vi "nanocal -- nuclear schottky fit -- 2x2 -- V9.vi"() -> ()   [LabVIEW 2021] (continued)
τC\" -> 0.001114108457   ,  \"κ0\" -> 0.000000000764   ,  \"mm1\" -> 0.000205034245   ,  \"mm2\" -> 0.015217532140   ,  \"mm3\" -> 0.169293678338   ,  \"T\" -> 0.178000000000   ,  \"B\" -> 8.000000000000   ,  \"θ\" -> 90.000000000000   ,  \"Reoff\" -> -44930693.069306924900   ,  \"Imoff\" -> 0.000000000000   ,  \"στ1\" -> 0.007491304915   ,  \"στS\" -> 0.004191211320   ,  \"στN\" -> 0.000000000000    |>   , \r\"IDS0348_210906_RAW_cal__sam_\" ->   <|    \"ζ\" -> 0.135783247929   ,  \"τ1\" -> 0.037121050091   ,  \"τS\" -> 0.079201640502   ,  \"τN\" -> 0.079201640502   ,  \"τC\" -> 0.001474311209   ,  \"κ0\" -> 0.000000000894   ,  \"mm1\" -> 0.000173730712   ,  \"mm2\" -> 0.016810842330   ,  \"mm3\" -> 0.201522581240   ,  \"T\" -> 0.178000000000   ,  \"B\" -> 8.000000000000   ,  \"θ\" -> 90.000000000000   ,  \"Reoff\" -> -29680722.891566276600   ,  \"Imoff\" -> 0.000000000000   ,  \"στ1\" -> 0.000000000000   ,  \"στS\" -> 0.000000000000   ,  \"στN\" -> 0.000000000000    |>   , \r\"IDS0349_210906_RAW_cal__ref_\" ->   <|    \"ζ\" -> 0.190984000958   ,  \"τ1\" -> 0.032898392235   ,  \"τS\" -> 0.053015075726   ,  \"τN\" -> 0.036446539803   ,  \"τC\" -> 0.001170894868   ,  \"κ0\" -> 0.000000001035   ,  \"mm1\" -> 0.000184864342   ,  \"mm2\" -> 0.017107531018   ,  \"mm3\" -> 0.123324244538   ,  \"T\" -> 0.200000000000   ,  \"B\" -> 8.000000000000   ,  \"θ\" -> 90.000000000000   ,  \"Reoff\" -> -24207920.792079202800   ,  \"Imoff\" -> 0.000000000000   ,  \"στ1\" -> 0.007827965999   ,  \"στS\" -> 0.003040573624   ,  \"στN\" -> 0.000000000000    |>   , \r\"IDS0349_210906_RAW_cal__sam_\" ->   <|    \"ζ\" -> 0.113690190882   ,  \"τ1\" -> 0.032691214581   ,  \"τS\" -> 0.068786957350   ,  \"τN\" -> 0.048058332081   ,  \"τC\" -> 0.001613875480   ,  \"κ0\" -> 0.000000001156   ,  \"mm1\" -> 0.000161675745   ,  \"mm2\" -> 0.017372504664   ,  \"mm3\" -> 0.146900362342   ,  \"T\" -> 0.200000000000   ,  \"B\" -> 8.000000000000   ,  \"θ\" -> 90.000000000000   ,  \"Reoff\" -> -14590361.445783138300   ,  \"Imoff\" -> 0.000000000000   ,  \"στ1\" -> 0.000000000000   ,  \"στS\" -> 0.000000000000   ,  \"στN\" -> 0.000000000000    |>   , \r\"IDS0350_210906_RAW_cal__ref_\" ->   <|    \"ζ\" -> 0.117284187691   ,  \"τ1\" -> 0.026970666142   ,  \"τS\" -> 0.042347096729   ,  \"τN\" -> 0.016129848116   ,  \"τC\" -> 0.001330224146   ,  \"κ0\" -> 0.000000001350   ,  \"mm1\" -> 0.000136193348   ,  \"mm2\" -> 0.017132196816   ,  \"mm3\" -> 0.076367865944   ,  \"T\" -> 0.260000000000   ,  \"B\" -> 8.000000000000   ,  \"θ\" -> 90.000000000000   ,  \"Reoff\" -> -13846534.653465345500   ,  \"Imoff\" -> 0.000000000000   ,  \"στ1\" -> 0.008626446357   ,  \"στS\" -> 0.001916708788   ,  \"στN\" -> 0.000000000000    |>   , \r\"IDS0350_210906_RAW_cal__sam_\" ->   <|    \"ζ\" -> 0.071614468485   ,  \"τ1\" -> 0.024327525692   ,  \"τS\" -> 0.055056024171   ,  \"τN\" -> 0.019709093999   ,  \"τC\" -> 0.001754398678   ,  \"κ0\" -> 0.000000001497   ,  \"mm1\" -> 0.000114067222   ,  \"mm2\" -> 0.016460052715   ,  \"mm3\" -> 0.089627186802   ,  \"T\" -> 0.260000000000   ,  \"B\" -> 8.000000000000   ,  \"θ\" -> 90.000000000000   ,  \"Reoff\" -> -10063253.012048184900   ,  \"Imoff\" -> 0.000000000000   ,  \"στ1\" -> 0.000000000000   ,  \"στS\" -> 0.000000000000   ,  \"στN\" -> 0.000000000000    |>   , \r\"IDS0351_210906_RAW_cal__ref_\" ->   <|    \"ζ\" -> 0.080944960576   ,  \"τ1\" -> 0.020924370017   ,  \"τS\" -> 0.037011167707   ,  \"τN\" -> 0.007898683051   ,  \"τC\" -> 0.001560823327   ,  \"κ0\" -> 0.000000001762   ,  \"mm1\" -> 0.000112792747   ,  \"mm2\" -> 0.015713715797   ,  \"mm3\" -> 0.055203761657   ,  \"T\" -> 0.310000000000   ,  \"B\" -> 8.000000000000   ,  \"θ\" -> 90.000000000000   ,  \"Reoff\" -> -7470297.029702961450   ,  \"Imoff\" -> 0.000000000000   ,  \"στ1\" -> 0.010612052509   ,  \"στS\" -> 0.001485327080   ,  \"στN\" -> 0.000000000000    |>   , \r\"IDS0351_210906_RAW_cal__sam_\" ->   <|    \"ζ\" -> 0.049866383839   ,  \"τ1\" -> 0.023285662985   ,  \"τS\" -> 0.049370833464   ,  \"τN\" -> 0.009866658615   ,  \"τC\" -> 0.002153040267   ,  \"κ0\" -> 0.000000001928   ,  \"mm1\" -> 0.000098362318   ,  \"mm2\" -> 0.018063601956   ,  \"mm3\" -> 0.069468190575   ,  \"T\" -> 0.310000000000   ,  \"B\" -> 8.000000000000   ,  \"θ\" -> 90.000000000000   ,  \"Reoff\" -> -5536144.578313261270   ,  \"Imoff\" -> 0.000000000000   ,  \"στ1\" -> 0.000000000000   ,  \"στS\" -> 0.000000000000   ,  \"στN\" -> 0.000000000000    |>   , \r\"IDS0352_210906_RAW_cal__ref_\" ->   <|    \"ζ\" -> 0.059924344954   ,  \"τ1\" -> 0.020444284414   ,  \"τS\" -> 0.034342319161   ,  \"τN\" -> 0.004837568639   ,  \"τC\" -> 0.001951892428   ,  \"κ0\" -> 0.000000002109   ,  \"mm1\" -> 0.000105020639   ,  \"mm2\" -> 0.016539029426   ,  \"mm3\" -> 0.047279843688   ,  \"T\" -> 0.360000000000   ,  \"B\" -> 8.000000000000   ,  \"θ\" -> 90.000000000000   ,  \"Reoff\" -> -3485148.514851480720   ,  \"Imoff\" -> 0.000000000000   ,  \"στ1\" -> 0.016824807524   ,  \"στS\" -> 0.001463681226   ,  \"στN\" -> 0.000000000000    |>   , \r\"IDS0352_210906_RAW_cal__sam_\" ->   <|    \"ζ\" -> 0.036116393265   ,  \"τ1\" -> 0.020310974732   ,  \"τS\" -> 0.044594628397   ,  \"τN\" -> 0.005932938101   ,  \"τC\" -> 0.002747123875   ,  \"κ0\" -> 0.000000002292   ,  \"mm1\" -> 0.000090548575   ,  \"mm2\" -> 0.017024776182   ,  \"mm3\" -> 0.058295213810   ,  \"T\" -> 0.360000000000   ,  \"B\" -> 8.000000000000   ,  \"θ\" -> 90.000000000000   ,  \"Reoff\" -> -2518072.289156645540   ,  \"Imoff\" -> 0.000000000000   ,  \"στ1\" -> 0.000000000000   ,  \"στS\" -> 0.000000000000   ,  \"στN\" -> 0.000000000000    |>   , \r\"IDS0353_210906_RAW_cal__ref_\" ->   <|    \"ζ\" -> 0.045101316453   ,  \"τ1\" -> 0.020505895958   ,  \"τS\" -> 0.031209032196   ,  \"τN\" -> 0.002683750708   ,  \"τC\" -> 0.002226651105   ,  \"κ0\" -> 0.000000002626   ,  \"mm1\" -> 0.000090181690   ,  \"mm2\" -> 0.017621773769   ,  \"mm3\" -> 0.040441983634   ,  \"T\" -> 0.438000000000   ,  \"B\" -> 8.000000000000   ,  \"θ\" -> 90.000000000000   ,  \"Reoff\" -> -2688118.811881184580   ,  \"Imoff\" -> 0.000000000000   ,  \"στ1\" -> 0.000000000000   ,  \"στS\" -> 0.000000000000   ,  \"στN\" -> 0.000000000000    |>   , \r\"IDS0353_210906_RAW_cal__sam_\" ->   <|    \"ζ\" -> 0.028235631162   ,  \"τ1\" -> 0.018033623612   ,  \"τS\" -> 0.040112967891   ,  \"τN\" -> 0.003332308168   ,  \"τC\" -> 0.002994357278   ,  \"κ0\" -> 0.000000002859   ,  \"mm1\" -> 0.000076791949   ,  \"mm2\" -> 0.016073609718   ,  \"mm3\" -> 0.049549560072   ,  \"T\" -> 0.438000000000   ,  \"B\" -> 8.000000000000   ,  \"θ\" -> 90.000000000000   ,  \"Reoff\" -> -2200000.000000000000   ,  \"Imoff\" -> 0.000000000000   ,  \"στ1\" -> 0.000000000000   ,  \"στS\" -> 0.000000000000   ,  \"στN\" -> 0.000000000000    |>   , \r\"IDS0354_210906_RAW_cal__ref_\" ->   <|    \"ζ\" -> 0.035449186867   ,  \"τ1\" -> 0.018569718484   ,  \"τS\" -> 0.028160564144   ,  \"τN\" -> 0.001513040869   ,  \"τC\" -> 0.002627412191   ,  \"κ0\" -> 0.000000003276   ,  \"mm1\" -> 0.000082729429   ,  \"mm2\" -> 0.016803631201   ,  \"mm3\" -> 0.035036280227   ,  \"T\" -> 0.530000000000   ,  \"B\" -> 8.000000000000   ,  \"θ\" -> 90.000000000000   ,  \"Reoff\" -> -2000000.000000000000   ,  \"Imoff\" -> 0.000000000000   ,  \"στ1\" -> 0.000000000000   ,  \"στS\" -> 0.000000000000   ,  \"στN\" -> 0.000000000000    |>   , \r\"IDS0354_210906_RAW_cal__sam_\" ->   <|    \"ζ\" -> 0.022962333090   ,  \"τ1\" -> 0.020865157142   ,  \"τS\" -> 0.035948400917   ,  \"τN\" -> 0.001990138096   ,  \"τC\" -> 0.003574397791   ,  \"κ0\" -> 0.000000003542   ,  \"mm1\" -> 0.000073258085   ,  \"mm2\" -> 0.019040364220   ,  \"mm3\" -> 0.044135629011   ,  \"T\" -> 0.530000000000   ,  \"B\" -> 8.000000000000   ,  \"θ\" -> 90.000000000000   ,  \"Reoff\" -> -1700000.000000000000   ,  \"Imoff\" -> 0.000000000000   ,  \"στ1\" -> 0.000000000000   ,  \"στS\" -> 0.000000000000   ,  \"στN\" -> 0.000000000000    |>   , \r\"IDS0355_210906_RAW_cal__ref_\" ->   <|    \"ζ\" -> 0.023121987816   ,  \"τ1\" -> 0.018681929200   ,  \"τS\" -> 0.017398280529   ,  \"τN\" -> 0.000397568997   ,  \"τC\" -> 0.004006240914   ,  \"κ0\" -> 0.000000005416   ,  \"mm1\" -> 0.000074156421   ,  \"mm2\" -> 0.017157833141   ,  \"mm3\" -> 0.023663505495   ,  \"T\" -> 0.830000000000   ,  \"B\" -> 8.000000000000   ,  \"θ\" -> 90.000000000000   ,  \"Reoff\" -> -695544.554455444216   ,  \"Imoff\" -> 0.000000000000   ,  \"στ1\" -> 0.000000000000   ,  \"στS\" -> 0.000000000000   ,  \"στN\" -> 0.000000000000    |>   , \r\"IDS0355_210906_RAW_cal__sam_\" ->   <|    \"ζ\" -> 0.015987398390   ,  \"τ1\" -> 0.023974349678   ,  \"τS\" -> 0.025824294014   ,  \"τN\" -> 0.000573136357   ,  \"τC\" -> 0.005688548480   ,  \"κ0\" -> 0.000000005865   ,  \"mm1\" -> 0.000073733721   ,  \"mm2\" -> 0.022561297233   ,  \"mm3\" -> 0.033847323811   ,  \"T\" -> 0.830000000000   ,  \"B\" -> 8.000000000000   ,  \"θ\" -> 90.000000000000   ,  \"Reoff\" -> -599999.999999999999   ,  \"Imoff\" -> 0.000000000000   ,  \"στ1\" -> 0.000000000000   ,  \"στS\" -> 0.000000000000   ,  \"στN\" -> 0.000000000000    |>   , \r\"IDS0359_210907_RAW_cal__ref_\" ->   <|    \"ζ\" -> 0.381969883498   ,  \"τ1\" -> 0.094329379305   ,  \"τS\" -> 0.076928325275   ,  \"τN\" -> 0.550887477218   ,  \"τC\" -> 0.001034779226   ,  \"κ0\" -> 0.000000000383   ,  \"mm1\" -> 0.000283958299   ,  \"mm2\" -> 0.010609033514   ,  \"mm3\" -> 0.952093698147   ,  \"T\" -> 0.120000000000   ,  \"B\" -> 12.000000000000   ,  \"θ\" -> 60.000000000000   ,  \"Reoff\" -> -100000000.000000000000   ,  \"Imoff\" -> 0.000000000000   ,  \"στ1\" -> 0.012489604376   ,  \"στS\" -> 0.015785658114   ,  \"στN\" -> 0.000000000000    |>   , \r\"IDS0359_210907_RAW_cal__sam_\" ->   <|    \"ζ\" -> 0.241762987309   ,  \"τ1\" -> 0.090301757431   ,  \"τS\" -> 0.104468976957   ,  \"τN\" -> 0.810352557873   ,  \"τC\" -> 0.001702208121   ,  \"κ0\" -> 0.000000000500   ,  \"mm1\" -> 0.000327834342   ,  \"mm2\" -> 0.009723084216   ,  \"mm3\" -> 1.217944568939   ,  \"T\" -> 0.120000000000   ,  \"B\" -> 12.000000000000   ,  \"θ\" -> 60.000000000000   ,  \"Reoff\" -> -52289156.626506023100   ,  \"Imoff\" -> 0.000000000000   ,  \"στ1\" -> 0.000000000000   ,  \"στS\" -> 0.000000000000   ,  \"στN\" -> 0.000000000000    |>   , \r\"IDS0360_210907_RAW_cal__ref_\" ->   <|    \"ζ\" -> 0.332032071502   ,  \"τ1\" -> 0.077785863829   ,  \"τS\" -> 0.054247117088   ,  \"τN\" -> 0.276531096522   ,  \"τC\" -> 0.001063816056   ,  \"κ0\" -> 0.000000000641   ,  \"mm1\" -> 0.000262214679   ,  \"mm2\" -> 0.011189186969   ,  \"mm3\" -> 0.508005467320   ,  \"T\" -> 0.150000000000   ,  \"B\" -> 12.000000000000   ,  \"θ\" -> 60.000000000000   ,  \"Reoff\" -> -64885542.168674700000   ,  \"Imoff\" -> 0.000000000000   ,  \"στ1\" -> 0.010441701195   ,  \"στS\" -> 0.005858449647   ,  \"στN\" -> 0.000000000000    |>   , \r\"IDS0360_210907_RAW_cal__sam_\" ->   <|    \"ζ\" -> 0.201278537585   ,  \"τ1\" -> 0.081544073952   ,  \"τS\" -> 0.088995303529   ,  \"τN\" -> 0.405130496924   ,  \"τC\" -> 0.001460686320   ,  \"κ0\" -> 0.000000000739   ,  \"mm1\" -> 0.000241947199   ,  \"mm2\" -> 0.013299947862   ,  \"mm3\" -> 0.663045584163   ,  \"T\" -> 0.150000000000   ,  \"B\" -> 12.000000000000   ,  \"θ\" -> 60.000000000000   ,  \"Reoff\" -> -39048192.771084338400   ,  \"Imoff\" -> 0.000000000000   ,  \"στ1\" -> 0.000000000000   ,  \"στS\" -> 0.000000000000   ,  \"στN\" -> 0.000000000000    |>   , \r\"IDS0361_210908_RAW_cal__ref_\" ->   <|    \"ζ\" -> 0.279785391024   ,  \"τ1\" -> 0.067061821351   ,  \"τS\" -> 0.048033272534   ,  \"τN\" -> 0.170024512607   ,  \"τC\" -> 0.001016043022   ,  \"κ0\" -> 0.000000000755   ,  \"mm1\" -> 0.000219251026   ,  \"mm2\" -> 0.012488143188   ,  \"mm3\" -> 0.334437637981   ,  \"T\" -> 0.168000000000   ,  \"B\" -> 12.000000000000   ,  \"θ\" -> 60.000000000000   ,  \"Reoff\" -> -50271084.337349399900   ,  \"Imoff\" -> 0.000000000000   ,  \"στ1\" -> 0.007974659835   ,  \"στS\" -> 0.004537587745   ,  \"στN\" -> 0.000000000000    |>   , \r\"IDS0361_210908_RAW_cal__sam_\" ->   <|    \"ζ\" -> 0.166104690940   ,  \"τ1\" -> 0.071049175548   ,  \"τS\" -> 0.068661809155   ,  \"τN\" -> 0.222482953546   ,  \"τC\" -> 0.001364223445   ,  \"κ0\" -> 0.000000000861   ,  \"mm1\" -> 0.000191495940   ,  \"mm2\" -> 0.014533832786   ,  \"mm3\" -> 0.397193343795   ,  \"T\" -> 0.168000000000   ,  \"B\" -> 12.000000000000   ,  \"θ\" -> 60.000000000000   ,  \"Reoff\" -> -34789156.626506023100   ,  \"Imoff\" -> 0.000000000000   ,  \"στ1\" -> 0.000000000000   ,  \"στS\" -> 0.000000000000   ,  \"στN\" -> 0.000000000000    |>   , \r\"IDS0362_210908_RAW_cal__ref_\" ->   <|    \"ζ\" -> 0.207142334401   ,  \"τ1\" -> 0.057894480183   ,  \"τS\" -> 0.038690220204   ,  \"τN\" -> 0.092417014932   ,  \"τC\" -> 0.001098696065   ,  \"κ0\" -> 0.000000001038   ,  \"mm1\" -> 0.000184887893   ,  \"mm2\" -> 0.013547417032   ,  \"mm3\" -> 0.203525965202   ,  \"T\" -> 0.197000000000   ,  \"B\" -> 12.000000000000   ,  \"θ\" -> 60.000000000000   ,  \"Reoff\" -> -28512048.192771077200   ,  \"Imoff\" -> 0.000000000000   ,  \"στ1\" -> 0.006011065509   ,  \"στS\" -> 0.002598249147   ,  \"στN\" -> 0.000000000000    |>   , \r\"IDS0362_210908_RAW_cal__sam_\" ->   <|    \"ζ\" -> 0.123741217510   ,  \"τ1\" -> 0.059103977068   ,  \"τS\" -> 0.051096152058   ,  \"τN\" -> 0.122661863704   ,  \"τC\" -> 0.001502836172   ,  \"κ0\" -> 0.000000001149   ,  \"mm1\" -> 0.000161683871   ,  \"mm2\" -> 0.014394250129   ,  \"mm3\" -> 0.241309923424   ,  \"T\" -> 0.197000000000   ,  \"B\" -> 12.000000000000   ,  \"θ\" -> 60.000000000000   ,  \"Reoff\" -> -17448795.180722892300   ,  \"Imoff\" -> 0.000000000000   ,  \"στ1\" -> 0.000000000000   ,  \"στS\" -> 0.000000000000   ,  \"στN\" -> 0.000000000000    |>   , \r\"IDS0363_210908_RAW_cal__ref_\" ->   <|    \"ζ\" -> 0.123120408408   ,  \"τ1\" -> 0.041426792490   ,  \"τS\" -> 0.030611483740   ,  \"τN\" -> 0.033673862745   ,  \"τC\" -> 0.001247428044   ,  \"κ0\" -> 0.000000001354   ,  \"mm1\" -> 0.000132437169   ,  \"mm2\" -> 0.014700070997   ,  \"mm3\" -> 0.100041896966   ,  \"T\" -> 0.250000000000   ,  \"B\" -> 12.000000000000   ,  \"θ\" -> 60.000000000000   ,  \"Reoff\" -> -14912650.602409631000   ,  \"Imoff\" -> 0.000000000000   ,  \"στ1\" -> 0.005277736765   ,  \"στS\" -> 0.001423482809   ,  \"στN\" -> 0.000000000000    |>   , \r\"IDS0363_210908_RAW_cal__sam_\" ->   <|    \"ζ\" -> 0.074359211271   ,  \"τ1\" -> 0.044477620306   ,  \"τS\" -> 0.040449563551   ,  \"τN\" -> 0.044745540249   ,  \"τC\" -> 0.001712765821   ,  \"κ0\" -> 0.000000001493   ,  \"mm1\" -> 0.000114327803   ,  \"mm2\" -> 0.016556677808   ,  \"mm3\" -> 0.121049525039   ,  \"T\" -> 0.250000000000   ,  \"B\" -> 12.000000000000   ,  \"θ\" -> 60.000000000000   ,  \"Reoff\" -> -10147590.361445784600   ,  \"Imoff\" -> 0.000000000000   ,  \"στ1\" -> 0.000000000000   ,  \"στS\" -> 0.000000000000   ,  \"στN\" -> 0.000000000000    |>   , \r\"IDS0364_210908_RAW_cal__ref_\" ->   <|    \"ζ\" -> 0.083964366121   ,  \"τ1\" -> 0.035864566651   ,  \"τS\" -> 0.027410501881   ,  \"τN\" -> 0.017171198615   ,  \"τC\" -> 0.001554769636   ,  \"κ0\" -> 0.000000001739   ,  \"mm1\" -> 0.000114855748   ,  \"mm2\" -> 0.016061286678   ,  \"mm3\" -> 0.069568168580   ,  \"T\" -> 0.307000000000   ,  \"B\" -> 12.000000000000   ,  \"θ\" -> 60.000000000000   ,  \"Reoff\" -> -7659638.554216861730   ,  \"Imoff\" -> 0.000000000000   ,  \"στ1\" -> 0.006264566865   ,  \"στS\" -> 0.001087528836   ,  \"στN\" -> 0.000000000000    |>   , \r\"IDS0364_210908_RAW_cal__sam_\" ->   <|    \"ζ\" -> 0.051560123380   ,  \"τ1\" -> 0.037167172913   ,  \"τS\" -> 0.035875072163   ,  \"τN\" -> 0.021782945969   ,  \"τC\" -> 0.002191662682   ,  \"κ0\" -> 0.000000001902   ,  \"mm1\" -> 0.000101812126   ,  \"mm2\" -> 0.018093196790   ,  \"mm3\" -> 0.081794699340   ,  \"T\" -> 0.307000000000   ,  \"B\" -> 12.000000000000   ,  \"θ\" -> 60.000000000000   ,  \"Reoff\" -> -5584337.349397592250   ,  \"Imoff\" -> 0.000000000000   ,  \"στ1\" -> 0.000000000000   ,  \"στS\" -> 0.000000000000   ,  \"στN\" -> 0.000000000000    |>   , \r\"IDS0365_210908_RAW_cal__ref_\" ->   <|    \"ζ\" -> 0.061646569706   ,  \"τ1\" -> 0.029620794864   ,  \"τS\" -> 0.025192478366   ,  \"τN\" -> 0.009702290524   ,  \"τC\" -> 0.001914430909   ,  \"κ0\" -> 0.000000002114   ,  \"mm1\" -> 0.000104108758   ,  \"mm2\" -> 0.016173173755   ,  \"mm3\" -> 0.052303854953   ,  \"T\" -> 0.360000000000   ,  \"B\" -> 12.000000000000   ,  \"θ\" -> 60.000000000000   ,  \"Reoff\" -> -4033132.530120491980   ,  \"Imoff\" -> 0.000000000000   ,  \"στ1\" -> 0.007715852130   ,  \"στS\" -> 0.000971919235   ,  \"στN\" -> 0.000000000000    |>   , \r\"IDS0365_210908_RAW_cal__sam_\" ->   <|    \"ζ\" -> 0.037527154631   ,  \"τ1\" -> 0.031791574880   ,  \"τS\" -> 0.032568278603   ,  \"τN\" -> 0.012463984296   ,  \"τC\" -> 0.002682405917   ,  \"κ0\" -> 0.000000002306   ,  \"mm1\" -> 0.000090102201   ,  \"mm2\" -> 0.018466994147   ,  \"mm3\" -> 0.062639080041   ,  \"T\" -> 0.360000000000   ,  \"B\" -> 12.000000000000   ,  \"θ\" -> 60.000000000000   ,  \"Reoff\" -> -2846385.542168676850   ,  \"Imoff\" -> 0.000000000000   ,  \"στ1\" -> 0.000000000000   ,  \"στS\" -> 0.000000000000   ,  \"στN\" -> 0.000000000000    |>   , \r\"IDS0366_210908_RAW_cal__ref_\" ->   <|    \"ζ\" -> 0.045512932741   ,  \"τ1\" -> 0.026001941230   ,  \"τS\" -> 0.023139529347   ,  \"τN\" -> 0.005224117100   ,  \"τC\" -> 0.002327747283   ,  \"κ0\" -> 0.000000002647   ,  \"mm1\" -> 0.000092754843   ,  \"mm2\" -> 0.016672258116   ,  \"mm3\" -> 0.041219234735   ,  \"T\" -> 0.430000000000   ,  \"B\" -> 12.000000000000   ,  \"θ\" -> 60.000000000000   ,  \"Reoff\" -> -2219879.518072277310   ,  \"Imoff\" -> 0.000000000000   ,  \"στ1\" -> 0.011333887810   ,  \"στS\" -> 0.000897031833   ,  \"στN\" -> 0.000000000000    |>   , \r\"IDS0366_210908_RAW_cal__sam_\" ->   <|    \"ζ\" -> 0.029143715364   ,  \"τ1\" -> 0.026198855926   ,  \"τS\" -> 0.029745373312   ,  \"τN\" -> 0.006649011545   ,  \"τC\" -> 0.003090491846   ,  \"κ0\" -> 0.000000002869   ,  \"mm1\" -> 0.000079676072   ,  \"mm2\" -> 0.018163106475   ,  \"mm3\" -> 0.048501617675   ,  \"T\" -> 0.430000000000   ,  \"B\" -> 12.000000000000   ,  \"θ\" -> 60.000000000000   ,  \"Reoff\" -> -2237951.807228915390   ,  \"Imoff\" -> 0.000000000000   ,  \"στ1\" -> 0.000000000000   ,  \"στS\" -> 0.000000000000   ,  \"στN\" -> 0.000000000000    |>   , \r\"IDS0367_210908_RAW_cal__ref_\" ->   <|    \"ζ\" -> 0.037324451442   ,  \"τ1\" -> 0.019605264024   ,  \"τS\" -> 0.021700560504   ,  \"τN\" -> 0.002800944156   ,  \"τC\" -> 0.002526998509   ,  \"κ0\" -> 0.000000003301   ,  \"mm1\" -> 0.000082012466   ,  \"mm2\" -> 0.015132192259   ,  \"mm3\" -> 0.032334067689   ,  \"T\" -> 0.530000000000   ,  \"B\" -> 12.000000000000   ,  \"θ\" -> 60.000000000000   ,  \"Reoff\" -> 0.000000000000   ,  \"Imoff\" -> 0.000000000000   ,  \"στ1\" -> 0.000000000000   ,  \"στS\" -> 0.000000000000   ,  \"στN\" -> 0.000000000000    |>   , \r\"IDS0367_210908_RAW_cal__sam_\" ->   <|    \"ζ\" -> 0.024637271207   ,  \"τ1\" -> 0.025634847148   ,  \"τS\" -> 0.027302474030   ,  \"τN\" -> 0.003538185279   ,  \"τC\" -> 0.003933377133   ,  \"κ0\" -> 0.000000003566   ,  \"mm1\" -> 0.000083131278   ,  \"mm2\" -> 0.019726981228   ,  \"mm3\" -> 0.041358600771   ,  \"T\" -> 0.530000000000   ,  \"B\" -> 12.000000000000   ,  \"θ\" -> 60.000000000000   ,  \"Reoff\" -> -1629518.072289161380   ,  \"Imoff\" -> 0.000000000000   ,  \"στ1\" -> 0.000000000000   ,  \"στS\" -> 0.000000000000   ,  \"στN\" -> 0.000000000000    |>   , \r\"IDS0368_210908_RAW_cal__ref_\" ->   <|    \"ζ\" -> 0.030581023885   ,  \"τ1\" -> 0.017326525290   ,  \"τS\" -> 0.020225378130   ,  \"τN\" -> 0.001703135365   ,  \"τC\" -> 0.003380889395   ,  \"κ0\" -> 0.000000003914   ,  \"mm1\" -> 0.000086626446   ,  \"mm2\" -> 0.014628874360   ,  \"mm3\" -> 0.028591023770   ,  \"T\" -> 0.630000000000   ,  \"B\" -> 12.000000000000   ,  \"θ\" -> 60.000000000000   ,  \"Reoff\" -> 0.000000000000   ,  \"Imoff\" -> 0.000000000000   ,  \"στ1\" -> 0.000000000000   ,  \"στS\" -> 0.000000000000   ,  \"στN\" -> 0.000000000000    |>   , \r\"IDS0368_210908_RAW_cal__sam_\" ->   <|    \"ζ\" -> 0.021420270760   ,  \"τ1\" -> 0.018208454683   ,  \"τS\" -> 0.024985612374   ,  \"τN\" -> 0.002144760910   ,  \"τC\" -> 0.004931614434   ,  \"κ0\" -> 0.000000004254   ,  \"mm1\" -> 0.000086915042   ,  \"mm2\" -> 0.015826314138   ,  \"mm3\" -> 0.034938353162   ,  \"T\" -> 0.630000000000   ,  \"B\" -> 12.000000000000   ,  \"θ\" -> 60.000000000000   ,  \"Reoff\" -> -1204819.277108438310   ,  \"Imoff\" -> 0.000000000000   ,  \"στ1\" -> 0.000000000000   ,  \"στS\" -> 0.000000000000   ,  \"στN\" -> 0.000000000000    |>   , \r\"IDS0369_210908_RAW_cal__ref_\" ->   <|    \"ζ\" -> 0.022212344829   ,  \"τ1\" -> 0.017343641344   ,  \"τS\" -> 0.018001662092   ,  \"τN\" -> 0.000711569404   ,  \"τC\" -> 0.004309595418   ,  \"κ0\" -> 0.000000005439   ,  \"mm1\" -> 0.000076128819   ,  \"mm2\" -> 0.015699102017   ,  \"mm3\" -> 0.025006902173   ,  \"T\" -> 0.830000000000   ,  \"B\" -> 12.000000000000   ,  \"θ\" -> 60.000000000000   ,  \"Reoff\" -> 0.000000000000   ,  \"Imoff\" -> 0.000000000000   ,  \"στ1\" -> 0.000000000000   ,  \"στS\" -> 0.000000000000   ,  \"στN\" -> 0.000000000000    |>   , \r\"IDS0369_210908_RAW_cal__sam_\" ->   <|    \"ζ\" -> 0.014606512986   ,  \"τ1\" -> 0.019756664879   ,  \"τS\" -> 0.022303249954   ,  \"τN\" -> 0.001023812506   ,  \"τC\" -> 0.005490022400   ,  \"κ0\" -> 0.000000005866   ,  \"mm1\" -> 0.000063747249   ,  \"mm2\" -> 0.017921258799   ,  \"mm3\" -> 0.030929470731   ,  \"T\" -> 0.830000000000   ,  \"B\" -> 12.000000000000   ,  \"θ\" -> 60.000000000000   ,  \"Reoff\" -> -481927.710843376814   ,  \"Imoff\" -> 0.000000000000   ,  \"στ1\" -> 0.000000000000   ,  \"στS\" -> 0.000000000000   ,  \"στN\" -> 0.000000000000    |>   , \r\"IDS0370_210908_RAW_cal__ref_\" ->   <|    \"ζ\" -> 0.021569402950   ,  \"τ1\" -> 0.017921737944   ,  \"τS\" -> 0.015463128015   ,  \"τN\" -> 0.000390873619   ,  \"τC\" -> 0.004954240411   ,  \"κ0\" -> 0.000000007586   ,  \"mm1\" -> 0.000079935600   ,  \"mm2\" -> 0.016393641357   ,  \"mm3\" -> 0.022598364382   ,  \"T\" -> 1.130000000000   ,  \"B\" -> 12.000000000000   ,  \"θ\" -> 60.000000000000   ,  \"Reoff\" -> 0.000000000000   ,  \"Imoff\" -> 0.000000000000   ,  \"στ1\" -> 0.000000000000   ,  \"στS\" -> 0.000000000000   ,  \"στN\" -> 0.000000000000    |>   , \r\"IDS0370_210908_RAW_cal__sam_\" ->   <|    \"ζ\" -> 0.013427569249   ,  \"τ1\" -> 0.019934074843   ,  \"τS\" -> 0.019524726442   ,  \"τN\" -> 0.000513623253   ,  \"τC\" -> 0.005657316251   ,  \"κ0\" -> 0.000000008143   ,  \"mm1\" -> 0.000058424467   ,  \"mm2\" -> 0.018528796956   ,  \"mm3\" -> 0.027311585694   ,  \"T\" -> 1.130000000000   ,  \"B\" -> 12.000000000000   ,  \"θ\" -> 60.000000000000   ,  \"Reoff\" -> -481927.710843376814   ,  \"Imoff\" -> 0.000000000000   ,  \"στ1\" -> 0.000000000000   ,  \"στS\" -> 0.000000000000   ,  \"στN\" -> 0.000000000000    |>   , \r\"IDS0371_210908_RAW_cal__ref_\" ->   <|    \"ζ\" -> 0.020664849580   ,  \"τ1\" -> 0.018108723176   ,  \"τS\" -> 0.010299896170   ,  \"τN\" -> 0.000079818017   ,  \"τC\" -> 0.006259144045   ,  \"κ0\" -> 0.000000013130   ,  \"mm1\" -> 0.000079811267   ,  \"mm2\" -> 0.016056535433   ,  \"mm3\" -> 0.018825729941   ,  \"T\" -> 1.900000000000   ,  \"B\" -> 12.000000000000   ,  \"θ\" -> 60.000000000000   ,  \"Reoff\" -> 0.000000000000   ,  \"Imoff\" -> 0.000000000000   ,  \"στ1\" -> 0.000000000000   ,  \"στS\" -> 0.000000000000   ,  \"στN\" -> 0.000000000000    |>   , \r\"IDS0371_210908_RAW_cal__sam_\" ->   <|    \"ζ\" -> 0.009645933094   ,  \"τ1\" -> 0.020976887035   ,  \"τS\" -> 0.013140254521   ,  \"τN\" -> 0.000215522697   ,  \"τC\" -> 0.007317042194   ,  \"κ0\" -> 0.000000013897   ,  \"mm1\" -> 0.000045154509   ,  \"mm2\" -> 0.018728618799   ,  \"mm3\" -> 0.023004762073   ,  \"T\" -> 1.900000000000   ,  \"B\" -> 12.000000000000   ,  \"θ\" -> 60.000000000000   ,  \"Reoff\" -> -120481.927710846066   ,  \"Imoff\" -> 0.000000000000   ,  \"στ1\" -> 0.000000000000   ,  \"στS\" -> 0.000000000000   ,  \"στN\" -> 0.000000000000    |>   , \r\"IDS0372_210908_RAW_cal__ref_\" ->   <|    \"ζ\" -> 0.021592146431   ,  \"τ1\" -> 0.018093446545   ,  \"τS\" -> 0.007071841556   ,  \"τN\" -> 0.000029085223   ,  \"τC\" -> 0.005341206531   ,  \"κ0\" -> 0.000000023517   ,  \"mm1\" -> 0.000065243548   ,  \"mm2\" -> 0.012435446609   ,  \"mm3\" -> 0.018188213949   ,  \"T\" -> 3.110000000000   ,  \"B\" -> 12.000000000000   ,  \"θ\" -> 60.000000000000   ,  \"Reoff\" -> 0.000000000000   ,  \"Imoff\" -> 0.000000000000   ,  \"στ1\" -> 0.000000000000   ,  \"στS\" -> 0.000000000000   ,  \"στN\" -> 0.000000000000    |>   , \r\"IDS0372_210908_RAW_cal__sam_\" ->   <|    \"ζ\" -> 0.010006554735   ,  \"τ1\" -> 0.021193289022   ,  \"τS\" -> 0.010059776467   ,  \"τN\" -> 0.000092737128   ,  \"τC\" -> 0.005619947239   ,  \"κ0\" -> 0.000000024358   ,  \"mm1\" -> 0.000035931477   ,  \"mm2\" -> 0.015490366222   ,  \"mm3\" -> 0.021541043840   ,  \"T\" -> 3.110000000000   ,  \"B\" -> 12.000000000000   ,  \"θ\" -> 60.000000000000   ,  \"Reoff\" -> -120481.927710846066   ,  \"Imoff\" -> 0.000000000000   ,  \"στ1\" -> 0.000000000000   ,  \"στS\" -> 0.000000000000   ,  \"στN\" -> 0.000000000000    |>   , \r\"IDS0373_210908_RAW_cal__ref_\" ->   <|    \"ζ\" -> 0.028148688120   ,  \"τ1\" -> 0.012706961955   ,  \"τS\" -> 0.003881518121   ,  \"τN\" -> 0.000007160132   ,  \"τC\" -> 0.004346615253   ,  \"κ0\" -> 0.000000058313   ,  \"mm1\" -> 0.000057355729   ,  \"mm2\" -> 0.008266435527   ,  \"mm3\" -> 0.012727925396   ,  \"T\" -> 5.750000000000   ,  \"B\" -> 12.000000000000   ,  \"θ\" -> 60.000000000000   ,  \"Reoff\" -> 0.000000000000   ,  \"Imoff\" -> 0.000000000000   ,  \"στ1\" -> 0.000000000000   ,  \"στS\" -> 0.000000000000   ,  \"στN\" -> 0.000000000000    |>   , \r\"IDS0373_210908_RAW_cal__sam_\" ->   <|    \"ζ\" -> 0.009383547393   ,  \"τ1\" -> 0.021616814113   ,  \"τS\" -> 0.006389723126   ,  \"τN\" -> 0.000031102862   ,  \"τC\" -> 0.004593168461   ,  \"κ0\" -> 0.000000059183   ,  \"mm1\" -> 0.000024995592   ,  \"mm2\" -> 0.010985466166   ,  \"mm3\" -> 0.021680596929   ,  \"T\" -> 5.750000000000   ,  \"B\" -> 12.000000000000   ,  \"θ\" -> 60.000000000000   ,  \"Reoff\" -> -40000.000000000000   ,  \"Imoff\" -> 0.000000000000   ,  \"στ1\" -> 0.000000000000   ,  \"στS\" -> 0.000000000000   ,  \"στN\" -> 0.000000000000    |>   , \r\"IDS0377_210909_RAW_cal__ref_\" ->   <|    \"ζ\" -> 0.218126190413   ,  \"τ1\" -> 0.079838021846   ,  \"τS\" -> 0.035132352739   ,  \"τN\" -> 0.027061454869   ,  \"τC\" -> 0.001090107541   ,  \"κ0\" -> 0.000000001041   ,  \"mm1\" -> 0.000191179094   ,  \"mm2\" -> 0.026924011586   ,  \"mm3\" -> 0.129572844636   ,  \"T\" -> 0.197000000000   ,  \"B\" -> 8.000000000000   ,  \"θ\" -> 0.000000000000   ,  \"Reoff\" -> -30325301.204819276900   ,  \"Imoff\" -> 0.000000000000   ,  \"στ1\" -> 0.015121325479   ,  \"στS\" -> 0.001580446534   ,  \"στN\" -> 0.000000000000    |>   , \r\"IDS0377_210909_RAW_cal__sam_\" ->   <|    \"ζ\" -> 0.135798490691   ,  \"τ1\" -> 0.079257563336   ,  \"τS\" -> 0.046440970443   ,  \"τN\" -> 0.031537801980   ,  \"τC\" -> 0.001434159670   ,  \"κ0\" -> 0.000000001166   ,  \"mm1\" -> 0.000167444282   ,  \"mm2\" -> 0.031002991367   ,  \"mm3\" -> 0.138089459380   ,  \"T\" -> 0.197000000000   ,  \"B\" -> 8.000000000000   ,  \"θ\" -> 0.000000000000   ,  \"Reoff\" -> -18665662.650602411500   ,  \"Imoff\" -> 0.000000000000   ,  \"στ1\" -> 0.000000000000   ,  \"στS\" -> 0.000000000000   ,  \"στN\" -> 0.000000000000    |>   , \r\"IDS0378_210909_RAW_cal__ref_\" ->   <|    \"ζ\" -> 0.444552800957   ,  \"τ1\" -> 0.128860115614   ,  \"τS\" -> 0.109021040284   ,  \"τN\" -> 0.152308696924   ,  \"τC\" -> 0.001224528567   ,  \"κ0\" -> 0.000000000394   ,  \"mm1\" -> 0.000374811046   ,  \"mm2\" -> 0.044053094938   ,  \"mm3\" -> 0.463161342054   ,  \"T\" -> 0.122000000000   ,  \"B\" -> 8.000000000000   ,  \"θ\" -> 0.000000000000   ,  \"Reoff\" -> -133680722.891566262000   ,  \"Imoff\" -> 0.000000000000   ,  \"στ1\" -> 0.037474122176   ,  \"στS\" -> 0.013209355673   ,  \"στN\" -> 0.000000000000    |>   , \r\"IDS0378_210909_RAW_cal__sam_\" ->   <|    \"ζ\" -> 0.261650469875   ,  \"τ1\" -> 0.181870145043   ,  \"τS\" -> 0.168113301561   ,  \"τN\" -> 0.186965229666   ,  \"τC\" -> 0.001543998203   ,  \"κ0\" -> 0.000000000530   ,  \"mm1\" -> 0.000318362571   ,  \"mm2\" -> 0.069029342513   ,  \"mm3\" -> 0.562051433928   ,  \"T\" -> 0.122000000000   ,  \"B\" -> 8.000000000000   ,  \"θ\" -> 0.000000000000   ,  \"Reoff\" -> -63674698.795180723100   ,  \"Imoff\" -> 0.000000000000   ,  \"στ1\" -> 0.000000000000   ,  \"στS\" -> 0.000000000000   ,  \"στN\" -> 0.000000000000    |>   , \r\"IDS0379_210909_RAW_cal__ref_\" ->   <|    \"ζ\" -> 0.358941818136   ,  \"τ1\" -> 0.106560472447   ,  \"τS\" -> 0.062750754933   ,  \"τN\" -> 0.083489698826   ,  \"τC\" -> 0.001109485369   ,  \"κ0\" -> 0.000000000627   ,  \"mm1\" -> 0.000290253427   ,  \"mm2\" -> 0.033675860334   ,  \"mm3\" -> 0.272436112171   ,  \"T\" -> 0.148000000000   ,  \"B\" -> 8.000000000000   ,  \"θ\" -> 0.000000000000   ,  \"Reoff\" -> -71123493.975903615400   ,  \"Imoff\" -> 0.000000000000   ,  \"στ1\" -> 0.022940419447   ,  \"στS\" -> 0.005727663556   ,  \"στN\" -> 0.000000000000    |>   , \r\"IDS0379_210909_RAW_cal__sam_\" ->   <|    \"ζ\" -> 0.225699737863   ,  \"τ1\" -> 0.105340283181   ,  \"τS\" -> 0.080581728797   ,  \"τN\" -> 0.103261234048   ,  \"τC\" -> 0.001367459466   ,  \"κ0\" -> 0.000000000745   ,  \"mm1\" -> 0.000248975261   ,  \"mm2\" -> 0.035515573270   ,  \"mm3\" -> 0.296279465482   ,  \"T\" -> 0.148000000000   ,  \"B\" -> 8.000000000000   ,  \"θ\" -> 0.000000000000   ,  \"Reoff\" -> -47870481.927710846100   ,  \"Imoff\" -> 0.000000000000   ,  \"στ1\" -> 0.000000000000   ,  \"στS\" -> 0.000000000000   ,  \"στN\" -> 0.000000000000    |>   , \r\"IDS0380_210909_RAW_cal__ref_\" ->   <|    \"ζ\" -> 0.288906167077   ,  \"τ1\" -> 0.085305830839   ,  \"τS\" -> 0.050470435451   ,  \"τN\" -> 0.055834761417   ,  \"τC\" -> 0.001016000241   ,  \"κ0\" -> 0.000000000740   ,  \"mm1\" -> 0.000224990907   ,  \"mm2\" -> 0.028925222390   ,  \"mm3\" -> 0.194189041618   ,  \"T\" -> 0.168000000000   ,  \"B\" -> 8.000000000000   ,  \"θ\" -> 0.000000000000   ,  \"Reoff\" -> -51177710.843373492400   ,  \"Imoff\" -> 0.000000000000   ,  \"στ1\" -> 0.012964547595   ,  \"στS\" -> 0.003391652117   ,  \"στN\" -> 0.000000000000    |>   , \r\"IDS0380_210909_RAW_cal__sam_\" ->   <|    \"ζ\" -> 0.175751625392   ,  \"τ1\" -> 0.093635045165   ,  \"τS\" -> 0.061160146348   ,  \"τN\" -> 0.068664853746   ,  \"τC\" -> 0.001317909381   ,  \"κ0\" -> 0.000000000855   ,  \"mm1\" -> 0.000193962663   ,  \"mm2\" -> 0.031705338902   ,  \"mm3\" -> 0.215695607858   ,  \"T\" -> 0.168000000000   ,  \"B\" -> 8.000000000000   ,  \"θ\" -> 0.000000000000   ,  \"Reoff\" -> -37527108.433734938500   ,  \"Imoff\" -> 0.000000000000   ,  \"στ1\" -> 0.000000000000   ,  \"στS\" -> 0.000000000000   ,  \"στN\" -> 0.000000000000    |>   , \r\"IDS0381_210909_RAW_cal__ref_\" ->   <|    \"ζ\" -> 0.126929215903   ,  \"τ1\" -> 0.058068597672   ,  \"τS\" -> 0.026924833357   ,  \"τN\" -> 0.010980626621   ,  \"τC\" -> 0.001220007823   ,  \"κ0\" -> 0.000000001350   ,  \"mm1\" -> 0.000132654651   ,  \"mm2\" -> 0.023198783099   ,  \"mm3\" -> 0.078673938037   ,  \"T\" -> 0.250000000000   ,  \"B\" -> 8.000000000000   ,  \"θ\" -> 0.000000000000   ,  \"Reoff\" -> -15819277.108433738400   ,  \"Imoff\" -> 0.000000000000   ,  \"στ1\" -> 0.015255137459   ,  \"στS\" -> 0.000926224863   ,  \"στN\" -> 0.000000000000    |>   , \r\"IDS0381_210909_RAW_cal__sam_\" ->   <|    \"ζ\" -> 0.077362618852   ,  \"τ1\" -> 0.058638638627   ,  \"τS\" -> 0.035602410157   ,  \"τN\" -> 0.012932252536   ,  \"τC\" -> 0.001722606032   ,  \"κ0\" -> 0.000000001497   ,  \"mm1\" -> 0.000118727642   ,  \"mm2\" -> 0.027585733079   ,  \"mm3\" -> 0.084946215242   ,  \"T\" -> 0.250000000000   ,  \"B\" -> 8.000000000000   ,  \"θ\" -> 0.000000000000   ,  \"Reoff\" -> -9843373.493975907570   ,  \"Imoff\" -> 0.000000000000   ,  \"στ1\" -> 0.000000000000   ,  \"στS\" -> 0.000000000000   ,  \"στN\" -> 0.000000000000    |>   , \r\"IDS0382_210909_RAW_cal__ref_\" ->   <|    \"ζ\" -> 0.087213265729   ,  \"τ1\" -> 0.047168857768   ,  \"τS\" -> 0.024342516225   ,  \"τN\" -> 0.005605032155   ,  \"τC\" -> 0.001527723897   ,  \"κ0\" -> 0.000000001731   ,  \"mm1\" -> 0.000116341877   ,  \"mm2\" -> 0.022377768321   ,  \"mm3\" -> 0.058761843342   ,  \"T\" -> 0.300000000000   ,  \"B\" -> 8.000000000000   ,  \"θ\" -> 0.000000000000   ,  \"Reoff\" -> -7659638.554216861730   ,  \"Imoff\" -> 0.000000000000   ,  \"στ1\" -> 0.020347835445   ,  \"στS\" -> 0.000812834930   ,  \"στN\" -> 0.000000000000    |>   , \r\"IDS0382_210909_RAW_cal__sam_\" ->   <|    \"ζ\" -> 0.054029770351   ,  \"τ1\" -> 0.051440847518   ,  \"τS\" -> 0.032079834642   ,  \"τN\" -> 0.007150632998   ,  \"τC\" -> 0.002202148776   ,  \"κ0\" -> 0.000000001884   ,  \"mm1\" -> 0.000106291219   ,  \"mm2\" -> 0.027352636275   ,  \"mm3\" -> 0.067534149597   ,  \"T\" -> 0.300000000000   ,  \"B\" -> 8.000000000000   ,  \"θ\" -> 0.000000000000   ,  \"Reoff\" -> 0.000000000000   ,  \"Imoff\" -> 0.000000000000   ,  \"στ1\" -> 0.000000000000   ,  \"στS\" -> 0.000000000000   ,  \"στN\" -> 0.000000000000    |>   , \r\"IDS0383_210910_RAW_cal__ref_\" ->   <|    \"ζ\" -> 0.061570309960   ,  \"τ1\" -> 0.048310722428   ,  \"τS\" -> 0.023792409980   ,  \"τN\" -> 0.003687374315   ,  \"τC\" -> 0.001764707006   ,  \"κ0\" -> 0.000000002103   ,  \"mm1\" -> 0.000096006795   ,  \"mm2\" -> 0.023284907275   ,  \"mm3\" -> 0.055866238496   ,  \"T\" -> 0.360000000000   ,  \"B\" -> 8.000000000000   ,  \"θ\" -> 0.000000000000   ,  \"Reoff\" -> -3448979.591836734680   ,  \"Imoff\" -> 0.000000000000   ,  \"στ1\" -> 0.005347956996   ,  \"στS\" -> 0.000064354371   ,  \"στN\" -> 0.000271676879    |>   , \r\"IDS0383_210910_RAW_cal__sam_\" ->   <|    \"ζ\" -> 0.038341835326   ,  \"τ1\" -> 0.050866858713   ,  \"τS\" -> 0.030652081909   ,  \"τN\" -> 0.004623805952   ,  \"τC\" -> 0.002823684758   ,  \"κ0\" -> 0.000000002289   ,  \"mm1\" -> 0.000096034779   ,  \"mm2\" -> 0.028459102290   ,  \"mm3\" -> 0.061763836547   ,  \"T\" -> 0.360000000000   ,  \"B\" -> 8.000000000000   ,  \"θ\" -> 0.000000000000   ,  \"Reoff\" -> 0.000000000000   ,  \"Imoff\" -> 0.000000000000   ,  \"στ1\" -> 0.000000000000   ,  \"στS\" -> 0.000000000000   ,  \"στN\" -> 0.000000000000    |>   , \r\"IDS0384_210910_RAW_cal__ref_\" ->   <|    \"ζ\" -> 0.047202777788   ,  \"τ1\" -> 0.057863954153   ,  \"τS\" -> 0.024260411824   ,  \"τN\" -> 0.002654470453   ,  \"τC\" -> 0.001761397108   ,  \"κ0\" -> 0.000000002620   ,  \"mm1\" -> 0.000074450881   ,  \"mm2\" -> 0.024981139493   ,  \"mm3\" -> 0.062755100371   ,  \"T\" -> 0.430000000000   ,  \"B\" -> 8.000000000000   ,  \"θ\" -> 0.000000000000   ,  \"Reoff\" -> -3244897.959183673380   ,  \"Imoff\" -> 0.000000000000   ,  \"στ1\" -> 0.002290219569   ,  \"στS\" -> 0.000142046978   ,  \"στN\" -> 0.000047451996    |>   , \r\"IDS0384_210910_RAW_cal__sam_\" ->   <|    \"ζ\" -> 0.029950572027   ,  \"τ1\" -> 0.044923259835   ,  \"τS\" -> 0.030416367718   ,  \"τN\" -> 0.002541256331   ,  \"τC\" -> 0.003331031560   ,  \"κ0\" -> 0.000000002858   ,  \"mm1\" -> 0.000087776347   ,  \"mm2\" -> 0.029544080465   ,  \"mm3\" -> 0.052567158325   ,  \"T\" -> 0.430000000000   ,  \"B\" -> 8.000000000000   ,  \"θ\" -> 0.000000000000   ,  \"Reoff\" -> 0.000000000000   ,  \"Imoff\" -> 0.000000000000   ,  \"στ1\" -> 0.000000000000   ,  \"στS\" -> 0.000000000000   ,  \"στN\" -> 0.000000000000    |>   , \r\"IDS0385_210910_RAW_cal__ref_\" ->   <|    \"ζ\" -> 0.035475807726   ,  \"τ1\" -> 0.065760313158   ,  \"τS\" -> 0.025267783397   ,  \"τN\" -> 0.001609393203   ,  \"τC\" -> 0.002044840275   ,  \"κ0\" -> 0.000000003270   ,  \"mm1\" -> 0.000065128755   ,  \"mm2\" -> 0.026984383918   ,  \"mm3\" -> 0.068586306909   ,  \"T\" -> 0.530000000000   ,  \"B\" -> 8.000000000000   ,  \"θ\" -> 0.000000000000   ,  \"Reoff\" -> -1979591.836734693500   ,  \"Imoff\" -> 0.000000000000   ,  \"στ1\" -> 0.001664351640   ,  \"στS\" -> 0.000128238795   ,  \"στN\" -> 0.000017678335    |>   , \r\"IDS0385_210910_RAW_cal__sam_\" ->   <|    \"ζ\" -> 0.024600756648   ,  \"τ1\" -> 0.043958236582   ,  \"τS\" -> 0.031312750224   ,  \"τN\" -> 0.001348105931   ,  \"τC\" -> 0.003635120795   ,  \"κ0\" -> 0.000000003548   ,  \"mm1\" -> 0.000078569164   ,  \"mm2\" -> 0.031960914170   ,  \"mm3\" -> 0.049018211972   ,  \"T\" -> 0.530000000000   ,  \"B\" -> 8.000000000000   ,  \"θ\" -> 0.000000000000   ,  \"Reoff\" -> 0.000000000000   ,  \"Imoff\" -> 0.000000000000   ,  \"στ1\" -> 0.000000000000   ,  \"στS\" -> 0.000000000000   ,  \"στN\" -> 0.000000000000    |>   , \r\"IDS0386_210910_RAW_cal__ref_\" ->   <|    \"ζ\" -> 0.027356022248   ,  \"τ1\" -> 0.074378310089   ,  \"τS\" -> 0.026934589252   ,  \"τN\" -> 0.001226970514   ,  \"τC\" -> 0.002640125038   ,  \"κ0\" -> 0.000000003880   ,  \"mm1\" -> 0.000064313303   ,  \"mm2\" -> 0.029422406274   ,  \"mm3\" -> 0.076463663571   ,  \"T\" -> 0.630000000000   ,  \"B\" -> 8.000000000000   ,  \"θ\" -> 0.000000000000   ,  \"Reoff\" -> -918367.346938774919   ,  \"Imoff\" -> 0.000000000000   ,  \"στ1\" -> 0.006379756107   ,  \"στS\" -> 0.000121793583   ,  \"στN\" -> 0.000037562843    |>   , \r\"IDS0386_210910_RAW_cal__sam_\" ->   <|    \"ζ\" -> 0.019494767421   ,  \"τ1\" -> 0.040349410363   ,  \"τS\" -> 0.033202805363   ,  \"τN\" -> 0.000770756985   ,  \"τC\" -> 0.004303152006   ,  \"κ0\" -> 0.000000004241   ,  \"mm1\" -> 0.000073144130   ,  \"mm2\" -> 0.033928832906   ,  \"mm3\" -> 0.045286454378   ,  \"T\" -> 0.630000000000   ,  \"B\" -> 8.000000000000   ,  \"θ\" -> 0.000000000000   ,  \"Reoff\" -> 0.000000000000   ,  \"Imoff\" -> 0.000000000000   ,  \"στ1\" -> 0.000000000000   ,  \"στS\" -> 0.000000000000   ,  \"στN\" -> 0.000000000000    |>   , \r\"IDS0387_210910_RAW_cal__ref_\" ->   <|    \"ζ\" -> 0.019264160163   ,  \"τ1\" -> 0.087527894663   ,  \"τS\" -> 0.031057035415   ,  \"τN\" -> 0.000427139586   ,  \"τC\" -> 0.003758266843   ,  \"κ0\" -> 0.000000005420   ,  \"mm1\" -> 0.000063607457   ,  \"mm2\" -> 0.035059135271   ,  \"mm3\" -> 0.088254109969   ,  \"T\" -> 0.830000000000   ,  \"B\" -> 8.000000000000   ,  \"θ\" -> 0.000000000000   ,  \"Reoff\" -> -265306.122448978945   ,  \"Imoff\" -> 0.000000000000   ,  \"στ1\" -> 0.002293859023   ,  \"στS\" -> 0.000111457645   ,  \"στN\" -> 0.000005341576    |>   , \r\"IDS0387_210910_RAW_cal__sam_\" ->   <|    \"ζ\" -> 0.013958531253   ,  \"τ1\" -> 0.040449551738   ,  \"τS\" -> 0.038075316972   ,  \"τN\" -> 0.000218997482   ,  \"τC\" -> 0.005348147372   ,  \"κ0\" -> 0.000000005866   ,  \"mm1\" -> 0.000064761782   ,  \"mm2\" -> 0.038768935960   ,  \"mm3\" -> 0.045792848207   ,  \"T\" -> 0.830000000000   ,  \"B\" -> 8.000000000000   ,  \"θ\" -> 0.000000000000   ,  \"Reoff\" -> 0.000000000000   ,  \"Imoff\" -> 0.000000000000   ,  \"στ1\" -> 0.000000000000   ,  \"στS\" -> 0.000000000000   ,  \"στN\" -> 0.000000000000    |>   , \r\"IDS0388_210910_RAW_cal__ref_\" ->   <|    \"ζ\" -> 0.016281760718   ,  \"τ1\" -> 0.090583957743   ,  \"τS\" -> 0.040861551341   ,  \"τN\" -> 0.000285855584   ,  \"τC\" -> 0.003366386849   ,  \"κ0\" -> 0.000000007540   ,  \"mm1\" -> 0.000049943920   ,  \"mm2\" -> 0.044562023222   ,  \"mm3\" -> 0.091155736609   ,  \"T\" -> 1.130000000000   ,  \"B\" -> 8.000000000000   ,  \"θ\" -> 0.000000000000   ,  \"Reoff\" -> -428571.428571428172   ,  \"Imoff\" -> 0.000000000000   ,  \"στ1\" -> 0.001979710526   ,  \"στS\" -> 0.000154101040   ,  \"στN\" -> 0.000003400989    |>   , \r\"IDS0388_210910_RAW_cal__sam_\" ->   <|    \"ζ\" -> 0.011551866824   ,  \"τ1\" -> 0.040411227639   ,  \"τS\" -> 0.048181354691   ,  \"τN\" -> 0.000103559724   ,  \"τC\" -> 0.006232382617   ,  \"κ0\" -> 0.000000008161   ,  \"mm1\" -> 0.000063176601   ,  \"mm2\" -> 0.040126882627   ,  \"mm3\" -> 0.055296246344   ,  \"T\" -> 1.130000000000   ,  \"B\" -> 8.000000000000   ,  \"θ\" -> 0.000000000000   ,  \"Reoff\" -> 0.000000000000   ,  
